vi "Read configuration.vi"(8 "error in":errorcluster, 11 "DMM Channel":refnum<class "DMM Channel.lvclass">) -> (0 "error out":errorcluster, 2 "CEF_configuration":refnum<class "CEF_serializable configuration.lvclass">, 3 "DMM Channel out":refnum<class "DMM Channel.lvclass">)   [LabVIEW 2025, in "DMM.lvlib" / "DMM Channel.lvclass"]
doc: "Copyright 2017 National Instruments Corporation\n\nLicensed under the Apache License, Version 2.0 (the \"License\"); you may not use this file except in compliance with the License. You may obtain a copy of the License at http://www.apache.org/licenses/LICENSE-2.0\nUnless required by applicable law or agreed to in writing, software distributed under the License is distributed on an \"AS IS\" BASIS, WITHOUT WARRANTIES OR CONDITIONS OF ANY KIND, either express or implied. See the License for the specific language governing permissions and limitations under the License."
uses:
  DMM Channel.lvclass
  Users/Public/Documents/Sandia National Labs/TSS Plugin/CEF.lvlibp/serializable configuration/CEF_serializable configuration.lvclass
  DMM Channel.lvclass/DMM Channel.ctl
  Users/Public/Documents/Sandia National Labs/TSS Plugin/Abstract Engine.lvlibp/Channel configuration/Channel configuration.lvclass
  C:/Users/Public/Documents/Sandia National Labs/TSS Plugin/CEF.lvlibp/serializable configuration/CEF_serializable configuration.lvclass
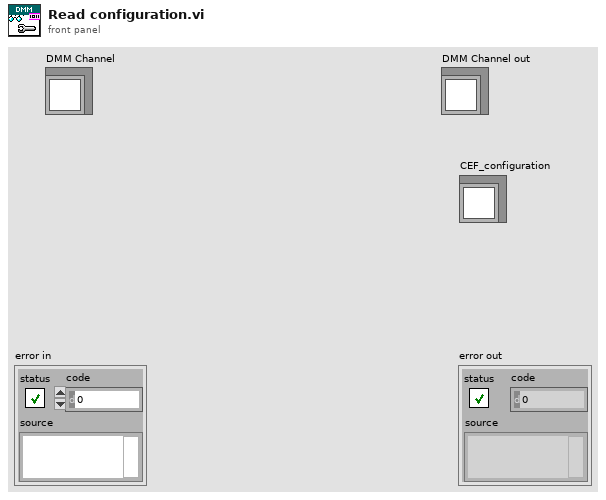
[diagram p1: front panel]
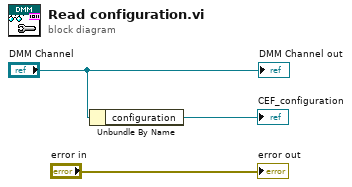
[diagram p0: block diagram]
diagram:
  n1 = Unbundle By Name("DMM Channel") -> ("configuration"=→"CEF_configuration":refnum<class "Channel configuration.lvclass">)
  "error out" <- "error in"
  "DMM Channel out" <- "DMM Channel"
